vi "Update Timestamp.vi"(7 "Timestamp":timestamp, 11 "Detection Frame In in":T1 {"robots_blue"."height" format="%+4.3f"; "robots_blue"."pixel_y" format="%+4.3f"; "robots_blue"."pixel_x" format="%+4.3f"; "robots_blue"."orientation" format="%+4.3f"; "robots_blue"."y" format="%+4.3f"; "robots_blue"."confidence" format="%4.3f"; "robots_blue"."x" format="%+4.3f"; "robots_yellow"."height" format="%+4.3f"; "robots_yellow"."pixel_y" format="%+4.3f"; "robots_yellow"."pixel_x" format="%+4.3f"; "robots_yellow"."orientation" format="%+4.3f"; "robots_yellow"."y" format="%+4.3f"; "robots_yellow"."confidence" format="%4.3f"; "robots_yellow"."x" format="%+4.3f"}) -> (3 "Detection Frame In out":T1 {"robots_blue"."height" format="%+4.3f"; "robots_blue"."pixel_y" format="%+4.3f"; "robots_blue"."pixel_x" format="%+4.3f"; "robots_blue"."orientation" format="%+4.3f"; "robots_blue"."y" format="%+4.3f"; "robots_blue"."confidence" format="%4.3f"; "robots_blue"."x" format="%+4.3f"; "robots_yellow"."height" format="%+4.3f"; "robots_yellow"."pixel_y" format="%+4.3f"; "robots_yellow"."pixel_x" format="%+4.3f"; "robots_yellow"."orientation" format="%+4.3f"; "robots_yellow"."y" format="%+4.3f"; "robots_yellow"."confidence" format="%4.3f"; "robots_yellow"."x" format="%+4.3f"})   [LabVIEW 2016]
uses:
  SSL Detection Frame.ctl
  SSL Detection Robot.ctl
  SSL Detection Ball.ctl
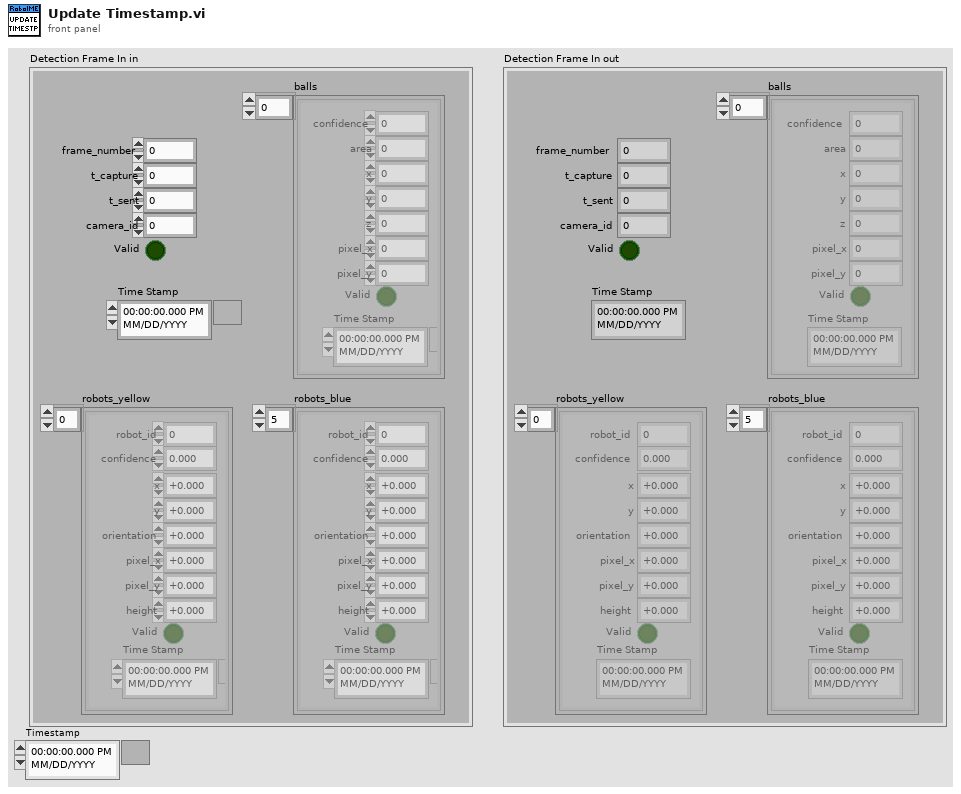
[diagram p1: front panel]
types:
  T1 = typedef "SSL Detection Frame.ctl" = cluster{"frame_number":u32, "t_capture":dbl, "t_sent":dbl, "camera_id":u32, "robots_yellow":T2[], "robots_blue":T2[], "balls":T3[], "Valid":bool, "Time Stamp":timestamp}
  T2 = typedef "SSL Detection Robot.ctl" = cluster{"x":sgl, "robot_id":u32, "confidence":sgl, "y":sgl, "orientation":sgl, "pixel_x":sgl, "pixel_y":sgl, "height":sgl, "Valid":bool, "Time Stamp":timestamp}
  T3 = typedef "SSL Detection Ball.ctl" = cluster{"x":sgl, "area":u32, "confidence":sgl, "y":sgl, "z":sgl, "pixel_x":sgl, "pixel_y":sgl, "Valid":bool, "Time Stamp":timestamp}
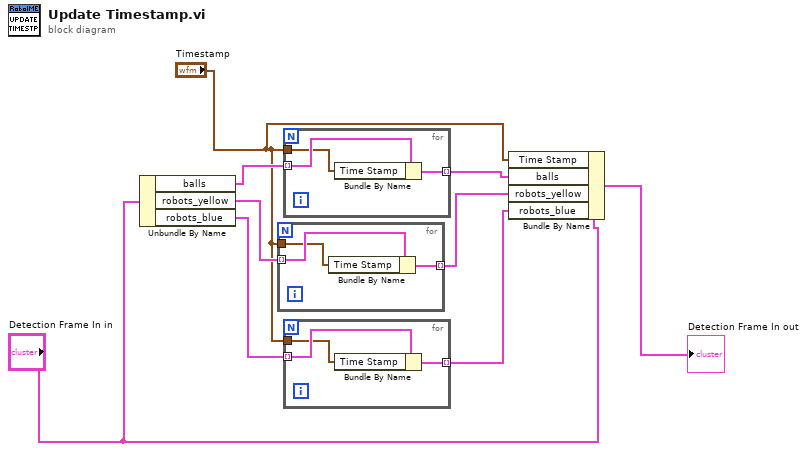
[diagram p0: block diagram]
diagram:
  n1 = Unbundle By Name("Detection Frame In in") -> ("balls"=w2:T3[], "robots_yellow"=w7:T2[], "robots_blue"=w9:T2[])
  n2 = for {
    tunnel: w7 -> [w12] mode=indexing
    tunnel: [w11] -> w5 mode=indexing
    tunnel: "Timestamp" -> [w10]
    n3 = Bundle By Name(cluster=w12, "Time Stamp"=w10) -> (w11:T2)
  }
  n4 = for {
    tunnel: w2 -> [w15] mode=indexing
    tunnel: [w14] -> w4 mode=indexing
    tunnel: "Timestamp" -> [w13]
    n5 = Bundle By Name(cluster=w15, "Time Stamp"=w13) -> (w14:T3)
  }
  n6 = for {
    tunnel: w9 -> [w18] mode=indexing
    tunnel: [w17] -> w6 mode=indexing
    tunnel: "Timestamp" -> [w16]
    n7 = Bundle By Name(cluster=w18, "Time Stamp"=w16) -> (w17:T2)
  }
  n8 = Bundle By Name(cluster="Detection Frame In in", "Time Stamp"="Timestamp", "balls"=w4, "robots_yellow"=w5, "robots_blue"=w6) -> (→"Detection Frame In out":T1)
